vi "Create castling move.vi"(4 "Rook destination":T1={"File"=enum."d", "Rank"=enum."4"}, 6 "Rook source":T1={"File"=enum."d", "Rank"=enum."4"}, 9 "Destination":T1={"File"=enum."d", "Rank"=enum."4"}, 10 "Source":T1={"File"=enum."d", "Rank"=enum."4"}) -> (3 "Castling out":refnum<class "Castling.lvclass">)   [LabVIEW 2015, in "Chesslib.lvlib" / "Castling.lvclass"]
uses:
  Castling.lvclass
  typedef/Square.ctl
  typedef/File.ctl
  typedef/Rank.ctl
  Pieces/King/King.lvclass
  Move/Move.lvclass/Move.ctl
  Castling.lvclass/Castling.ctl
  Move/Move.lvclass
  Chesslib.lvlib
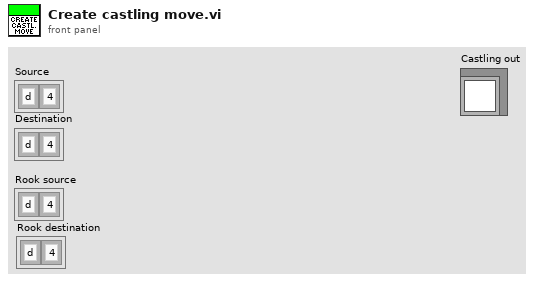
[diagram p1: front panel]
types:
  T1 = typedef "Chesslib.lvlib/Square.ctl" = cluster{"File":T2, "Rank":T3}
  T2 = typedef "Chesslib.lvlib/File.ctl" = enum8{"a", "b", "c", "d", "e", "f", "g", "h"}
  T3 = typedef "Chesslib.lvlib/Rank.ctl" = enum8{"1", "2", "3", "4", "5", "6", "7", "8"}
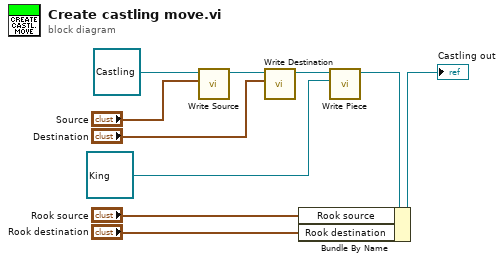
[diagram p0: block diagram]
diagram:
  n1 = call "Write Source.vi"("Square"="Source", "Move in"=refnum<class "Castling.lvclass"> refnum ("Castling in")) -> ("Move out"=w9:refnum<class "Castling.lvclass">)  [unwired: 8 in, 1 out]
  n2 = call "Write Destination.vi"("Square"="Destination", "Move in"=w9) -> ("Move out"=w4:refnum<class "Castling.lvclass">)  [unwired: 8 in, 1 out]
  n3 = call "Write Piece.vi"("Chesslib.lvlib:Piece.lvclass"=refnum<class "King.lvclass"> refnum ("Chesslib.lvlib:King.lvclass"), "Move in"=w4) -> ("Move out"=w2:refnum<class "Castling.lvclass">)  [unwired: 8 in, 1 out]
  n4 = Bundle By Name(cluster=w2, "Rook source"="Rook source", "Rook destination"="Rook destination") -> (→"Castling out":refnum<class "Castling.lvclass">)
